vi "VISA Serial Read (err silenced).vi"(4 "error in":errorcluster, 6 "byte count":u32, 7 "VISA resource name":refnum<visa-resource-name>) -> (0 "error IO":errorcluster, 1 "return count":u32, 2 "read buffer":string, 3 "VISA resource name out":refnum<visa-resource-name>)   [LabVIEW 2023]
doc: "Repackaged to eliminate description string in Error Cluster sent by read function whether there is an error or not."
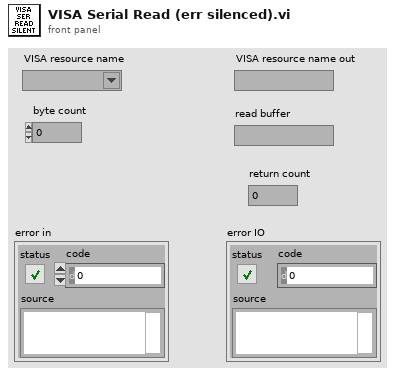
[diagram p1: front panel]
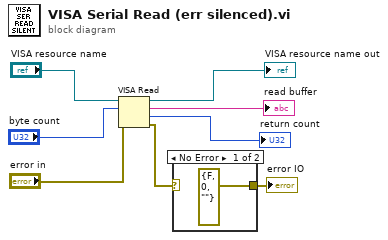
[diagram p0: block diagram]
diagram:
  n1 = VISA Read(VISA resource name="VISA resource name", byte count="byte count", error in (no error)="error in") -> (VISA resource name out=→"VISA resource name out":refnum<visa-resource-name>, read buffer=→"read buffer":string, return count=→"return count":u32, error out=w5:errorcluster)
  n2 = case shown="No Error" w5 {
    selector: w5 -> [_ w10]
    tunnel: [errorcluster {"status"=FALSE, "code"=0, "source"=""} ("error in (no error)") w10] -> w4
    frame No Error {
    }
    frame Error {
    }
  }
  "error IO" <- w4
